vi "Configure Trigger Characteristics.vi"(6 "Enable High Frequency Filter (F: Disable)":bool, 7 "Sensitivity (0.1 V)":dbl=0.1, 8 "error in (no error)":errorcluster, 9 "Trigger Holdoff (1E-7 s)":dbl=1e-07, 10 "Trigger Coupling (0: DC)":u16(ring) items=["DC", "AC", "Low Frequency Reject"], 11 "VISA resource name":refnum<visa-resource-name>) -> (0 "error out":errorcluster, 3 "VISA resource name out":refnum<visa-resource-name>)   [LabVIEW 2010, in "Agilent DSO1000 Series.lvlib"]
doc: "Configures trigger coupling, holdoff, sensitivty and high frequency filters."
uses:
  <instrlib>/Agilent DSO1000 Series/Agilent DSO1000 Series.lvlib
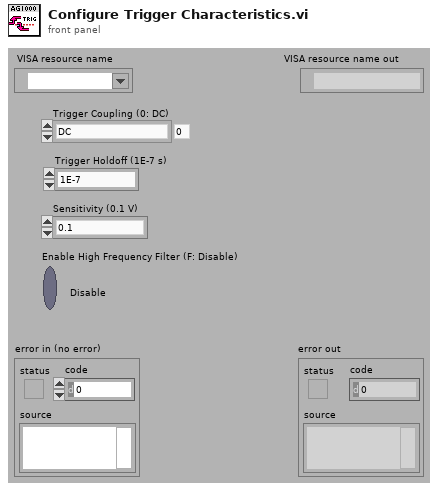
[diagram p1: front panel]
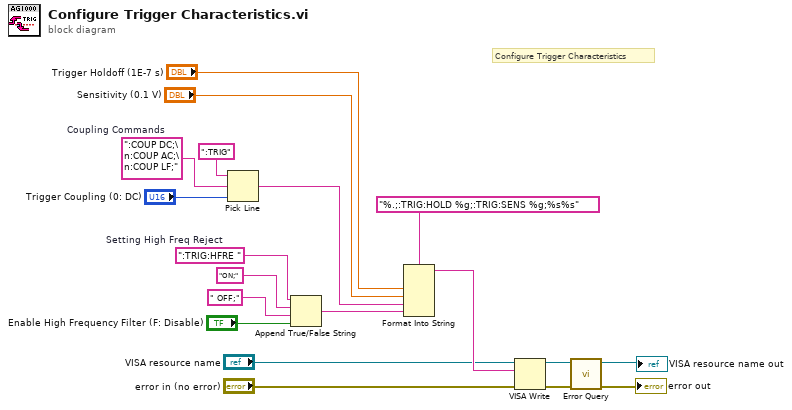
[diagram p0: block diagram]
diagram:
  w10 = ":TRIG:HFRE "  # Setting High Freq Reject
  w18 = ":COUP DC;\n:COUP AC;\n:COUP LF;"  # Coupling Commands
  # "Configure Trigger Characteristics"
  n1 = Pick Line(string ("")=":TRIG", multi-line string=w18, line index="Trigger Coupling (0: DC)") -> (output string=w5:string)
  n2 = Append True/False String(1:"Enable High Frequency Filter (F: Disable)", 2:" OFF;" ("string (\"\")"), 3:"ON;" ("Setting High Freq Reject"), 4:w10) -> (0:w4:string)
  n3 = Format Into String(format string="%.;:TRIG:HOLD %g;:TRIG:SENS %g;%s%s" ("Hold Off Command"), "Trigger Holdoff (1E-7 s)", "Sensitivity (0.1 V)", w5, w4) -> (resulting string=w3:string)  [unwired: 2 in, 1 out]
  n4 = VISA Write(VISA resource name="VISA resource name", write buffer=w3, error in (no error)="error in (no error)") -> (VISA resource name out=w14:refnum<visa-resource-name>, error out=w13:errorcluster)  [unwired: 1 out]
  n5 = call <instrlib>:"Error Query.vi"("error in (no error)"=w13, "VISA resource name"=w14) -> ("error out"=→"error out":errorcluster, "VISA resource name out"=→"VISA resource name out":refnum<visa-resource-name>)  [unwired: 6 in, 2 out]
